vi "F2-alle_sub.vi"(1 "% overtalk D-A":u8, 2 "% overtalk D-T2":u8, 3 "% overtalk D-T1":u8, 4 "binning (s)":refnum<vi>, 5 "Channel Akzeptor":refnum<vi>, 6 "HydraHarp":bool, 7 "Channel Transmitter2":refnum<vi>, 8 "Channel Transmitter1":refnum<vi>, 9 "Channel Donor":refnum<vi>) -> (0 "F2-Values":cluster{dbl, "Value":dbl, dbl[]}[](graph))   [LabVIEW 2009]
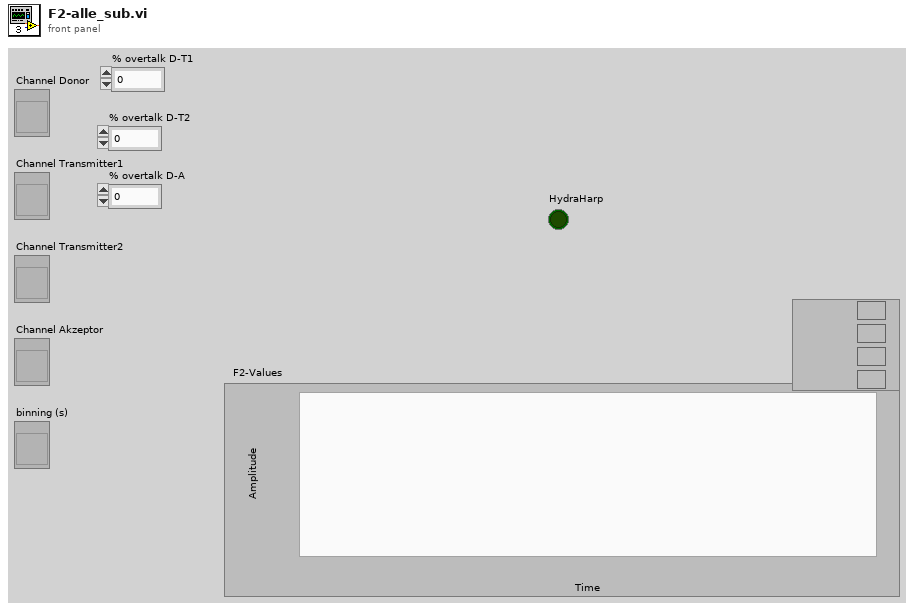
[diagram p1: front panel]
types:
  T1 = cluster{"router channels":u8[], "macro times":dbl[], "micro times":u16[], "invalid times":u32[], "gap times":u32[]}
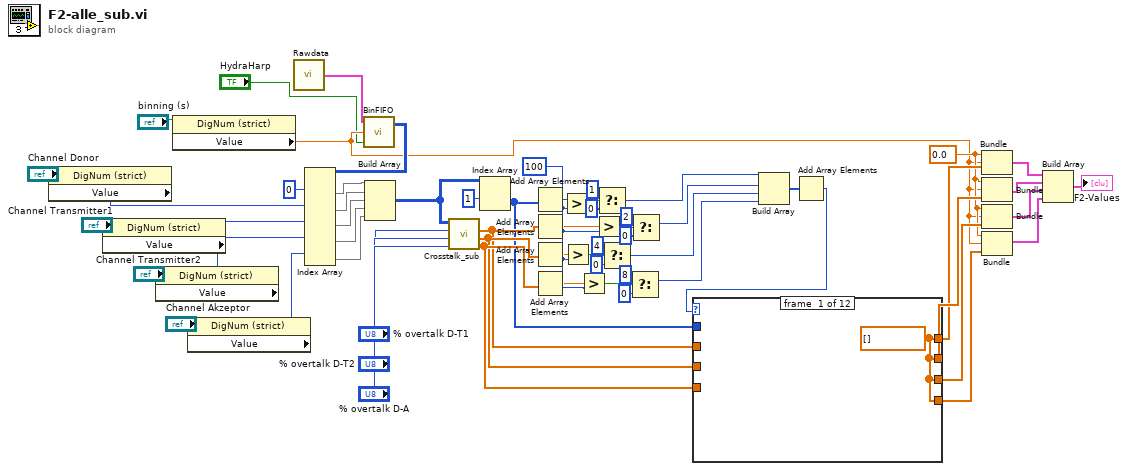
[diagram p0: block diagram]
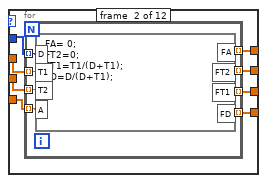
[diagram p2: hidden frame]
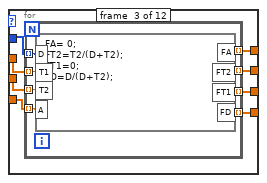
[diagram p3: hidden frame]
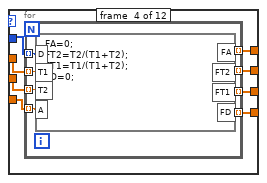
[diagram p4: hidden frame]
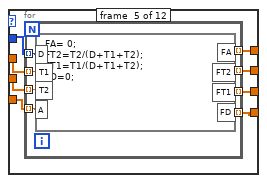
[diagram p5: hidden frame]
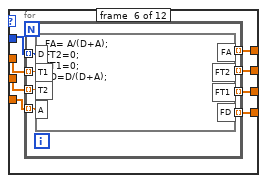
[diagram p6: hidden frame]
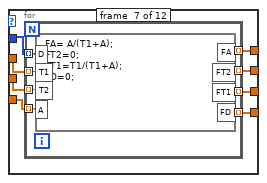
[diagram p7: hidden frame]
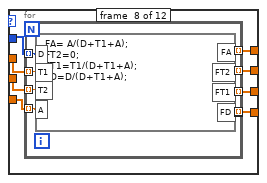
[diagram p8: hidden frame]
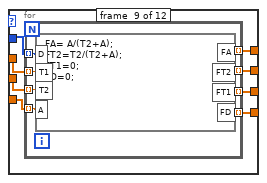
[diagram p9: hidden frame]
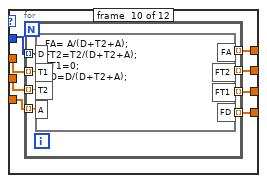
[diagram p10: hidden frame]
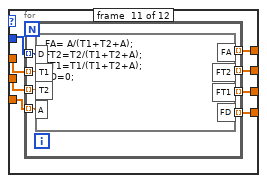
[diagram p11: hidden frame]
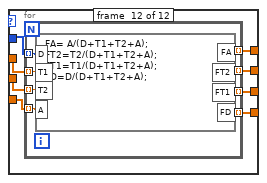
[diagram p12: hidden frame]
diagram:
  w22 = u16 100 ("y")
  w26 = 0.0
  n1 = property on="Property Node" class="DigNum (strict)"(reference="Channel Donor") -> ("Value"=w14:u8)  [unwired: 1 in, 2 out]
  n2 = property on="Property Node" class="DigNum (strict)"(reference="Channel Transmitter1") -> ("Value"=w15:u8)  [unwired: 1 in, 2 out]
  n3 = property on="Property Node" class="DigNum (strict)"(reference="Channel Transmitter2") -> ("Value"=w16:u8)  [unwired: 1 in, 2 out]
  n4 = property on="Property Node" class="DigNum (strict)"(reference="binning (s)") -> ("Value"=w6:dbl)  [unwired: 1 in, 2 out]
  n5 = property on="Property Node" class="DigNum (strict)"(reference="Channel Akzeptor") -> ("Value"=w17:u8)  [unwired: 1 in, 2 out]
  n6 = call "Rawdata.vi"() -> ("output rawdata"=w45:T1)  [unwired: 2 in]
  n7 = call "BinFIFO.vi"("HydraHarp"="HydraHarp", "binning (s)"=w6, "rawdata"=w45) -> ("MCS"=w18:u32[][])  [unwired: 1 out]
  n8 = Index Array(array=w18, index (row) #1=0 ("index (row)"), index (row) #2=w14, index (row) #3=w15, index (row) #4=w16, index (row) #5=w17) -> (element #1=w12:u32[], element #2=w11:u32[], element #3=w10:u32[], element #4=w9:u32[], element #5=w8:u32[])  [unwired: 5 in]
  n9 = Build Array(w12, w11, w10, w9, w8) -> (w7:u32[][])
  n10 = call "Crosstalk_sub.vi"("% overtalk D-T1"="% overtalk D-A", "% overtalk D-T2"="% overtalk D-T2", "% overtalk D-A"="% overtalk D-T1", "MCS_bg_corr"=w7) -> ("Akzeptor"=w5:dbl[], "Transmitter2"=w4:dbl[], "Transmitter1"=w3:dbl[])  [unwired: 1 out]
  n11 = Index Array(array=w7, index (row)=1) -> (element=w2:u32[])  [unwired: 1 in]
  n12 = Add Array Elements(numeric array=w2) -> (sum=w23:u32)
  n13 = Add Array Elements(numeric array=w3) -> (sum=w21:dbl)
  n14 = Add Array Elements(numeric array=w4) -> (sum=w20:dbl)
  n15 = Add Array Elements(numeric array=w5) -> (sum=w19:dbl)
  n16 = Greater?(x=w23, y=w22) -> (0:w44:bool)
  n17 = Greater?(x=w20, y=w22) -> (0:w35:bool)
  n18 = Greater?(x=w19, y=w22) -> (0:w41:bool)
  n19 = Greater?(x=w21, y=w22) -> (0:w38:bool)
  n20 = Select(t=u8 1, s=w44, f=u8 0) -> (s? t:f=w32:u8)
  n21 = Select(t=u8 4, s=w35, f=u8 0) -> (s? t:f=w30:u8)
  n22 = Select(t=u8 8, s=w41, f=u8 0) -> (s? t:f=w29:u8)
  n23 = Select(t=u8 2, s=w38, f=u8 0) -> (s? t:f=w31:u8)
  n24 = Build Array(w32, w31, w30, w29) -> (w28:u8[])
  n25 = Add Array Elements(numeric array=w28) -> (sum=w27:u8)
  n26 = case shown="11" w27 {
    tunnel: w2 -> [_ w70 w86 w102 w118 w134 w150 w166 w182 w198 w214 w230]
    tunnel: w3 -> [_ w69 w85 w101 w117 w133 w149 w165 w181 w197 w213 w229]
    tunnel: w4 -> [_ w68 w84 w100 w116 w132 w148 w164 w180 w196 w212 w228]
    tunnel: w5 -> [_ w67 w83 w99 w115 w131 w147 w163 w179 w195 w211 w227]
    tunnel: [w62 w66 w82 w98 w114 w130 w146 w162 w178 w194 w210 w226] -> w59
    tunnel: [w62 w65 w81 w97 w113 w129 w145 w161 w177 w193 w209 w225] -> w60
    tunnel: [w62 w64 w80 w96 w112 w128 w144 w160 w176 w192 w208 w224] -> w61
    tunnel: [w62 w63 w79 w95 w111 w127 w143 w159 w175 w191 w207 w223] -> w25
    frame #0 {
      w62 = dbl[] []
    }
    frame #1 {
      n27 = for {
        tunnel: w70 -> [w78] mode=indexing
        tunnel: w69 -> [w77] mode=indexing
        tunnel: w68 -> [w76] mode=indexing
        tunnel: w67 -> [w75] mode=indexing
        tunnel: [w74] -> w66 mode=indexing
        tunnel: [w73] -> w65 mode=indexing
        tunnel: [w72] -> w64 mode=indexing
        tunnel: [w71] -> w63 mode=indexing
        n28 = formula code="FA= 0;\nFT2=0;\nFT1=T1/(D+T1);\nFD=D/(D+T1);"("D"=w78, "T1"=w77, "T2"=w76, "A"=w75) -> ("FA"=w74:dbl, "FT2"=w73:dbl, "FT1"=w72:dbl, "FD"=w71:dbl)
      }
    }
    frame #2 {
      n29 = for {
        tunnel: w86 -> [w94] mode=indexing
        tunnel: w85 -> [w93] mode=indexing
        tunnel: w84 -> [w92] mode=indexing
        tunnel: w83 -> [w91] mode=indexing
        tunnel: [w90] -> w82 mode=indexing
        tunnel: [w89] -> w81 mode=indexing
        tunnel: [w88] -> w80 mode=indexing
        tunnel: [w87] -> w79 mode=indexing
        n30 = formula code="FA= 0;\nFT2=T2/(D+T2);\nFT1=0;\nFD=D/(D+T2);"("D"=w94, "T1"=w93, "T2"=w92, "A"=w91) -> ("FA"=w90:dbl, "FT2"=w89:dbl, "FT1"=w88:dbl, "FD"=w87:dbl)
      }
    }
    frame #3 {
      n31 = for {
        tunnel: w102 -> [w110] mode=indexing
        tunnel: w101 -> [w109] mode=indexing
        tunnel: w100 -> [w108] mode=indexing
        tunnel: w99 -> [w107] mode=indexing
        tunnel: [w106] -> w98 mode=indexing
        tunnel: [w105] -> w97 mode=indexing
        tunnel: [w104] -> w96 mode=indexing
        tunnel: [w103] -> w95 mode=indexing
        n32 = formula code="FA=0;\nFT2=T2/(T1+T2);\nFT1=T1/(T1+T2);\nFD=0;"("D"=w110, "T1"=w109, "T2"=w108, "A"=w107) -> ("FA"=w106:dbl, "FT2"=w105:dbl, "FT1"=w104:dbl, "FD"=w103:dbl)
      }
    }
    frame #4 {
      n33 = for {
        tunnel: w118 -> [w126] mode=indexing
        tunnel: w117 -> [w125] mode=indexing
        tunnel: w116 -> [w124] mode=indexing
        tunnel: w115 -> [w123] mode=indexing
        tunnel: [w122] -> w114 mode=indexing
        tunnel: [w121] -> w113 mode=indexing
        tunnel: [w120] -> w112 mode=indexing
        tunnel: [w119] -> w111 mode=indexing
        n34 = formula code="FA= 0;\nFT2=T2/(D+T1+T2);\nFT1=T1/(D+T1+T2);\nFD=0;"("D"=w126, "T1"=w125, "T2"=w124, "A"=w123) -> ("FA"=w122:dbl, "FT2"=w121:dbl, "FT1"=w120:dbl, "FD"=w119:dbl)
      }
    }
    frame #5 {
      n35 = for {
        tunnel: w134 -> [w142] mode=indexing
        tunnel: w133 -> [w141] mode=indexing
        tunnel: w132 -> [w140] mode=indexing
        tunnel: w131 -> [w139] mode=indexing
        tunnel: [w138] -> w130 mode=indexing
        tunnel: [w137] -> w129 mode=indexing
        tunnel: [w136] -> w128 mode=indexing
        tunnel: [w135] -> w127 mode=indexing
        n36 = formula code="FA= A/(D+A);\nFT2=0;\nFT1=0;\nFD=D/(D+A);"("D"=w142, "T1"=w141, "T2"=w140, "A"=w139) -> ("FA"=w138:dbl, "FT2"=w137:dbl, "FT1"=w136:dbl, "FD"=w135:dbl)
      }
    }
    frame #6 {
      n37 = for {
        tunnel: w150 -> [w158] mode=indexing
        tunnel: w149 -> [w157] mode=indexing
        tunnel: w148 -> [w156] mode=indexing
        tunnel: w147 -> [w155] mode=indexing
        tunnel: [w154] -> w146 mode=indexing
        tunnel: [w153] -> w145 mode=indexing
        tunnel: [w152] -> w144 mode=indexing
        tunnel: [w151] -> w143 mode=indexing
        n38 = formula code="FA= A/(T1+A);\nFT2=0;\nFT1=T1/(T1+A);\nFD=0;"("D"=w158, "T1"=w157, "T2"=w156, "A"=w155) -> ("FA"=w154:dbl, "FT2"=w153:dbl, "FT1"=w152:dbl, "FD"=w151:dbl)
      }
    }
    frame #7 {
      n39 = for {
        tunnel: w166 -> [w174] mode=indexing
        tunnel: w165 -> [w173] mode=indexing
        tunnel: w164 -> [w172] mode=indexing
        tunnel: w163 -> [w171] mode=indexing
        tunnel: [w170] -> w162 mode=indexing
        tunnel: [w169] -> w161 mode=indexing
        tunnel: [w168] -> w160 mode=indexing
        tunnel: [w167] -> _ mode=indexing
        tunnel: [w167] -> w159 mode=indexing
        n40 = formula code="FA= A/(D+T1+A);\nFT2=0;\nFT1=T1/(D+T1+A);\nFD=D/(D+T1+A);"("D"=w174, "T1"=w173, "T2"=w172, "A"=w171) -> ("FA"=w170:dbl, "FT2"=w169:dbl, "FT1"=w168:dbl, "FD"=w167:dbl)
      }
    }
    frame #8 {
      n41 = for {
        tunnel: w182 -> [w190] mode=indexing
        tunnel: w181 -> [w189] mode=indexing
        tunnel: w180 -> [w188] mode=indexing
        tunnel: w179 -> [w187] mode=indexing
        tunnel: [w186] -> w178 mode=indexing
        tunnel: [w185] -> w177 mode=indexing
        tunnel: [w184] -> w176 mode=indexing
        tunnel: [w183] -> w175 mode=indexing
        n42 = formula code="FA= A/(T2+A);\nFT2=T2/(T2+A);\nFT1=0;\nFD=0;"("D"=w190, "T1"=w189, "T2"=w188, "A"=w187) -> ("FA"=w186:dbl, "FT2"=w185:dbl, "FT1"=w184:dbl, "FD"=w183:dbl)
      }
    }
    frame #9 {
      n43 = for {
        tunnel: w198 -> [w206] mode=indexing
        tunnel: w197 -> [w205] mode=indexing
        tunnel: w196 -> [w204] mode=indexing
        tunnel: w195 -> [w203] mode=indexing
        tunnel: [w202] -> w194 mode=indexing
        tunnel: [w201] -> w193 mode=indexing
        tunnel: [w200] -> w192 mode=indexing
        tunnel: [w199] -> w191 mode=indexing
        n44 = formula code="FA= A/(D+T2+A);\nFT2=T2/(D+T2+A);\nFT1=0;\nFD=D/(D+T2+A);"("D"=w206, "T1"=w205, "T2"=w204, "A"=w203) -> ("FA"=w202:dbl, "FT2"=w201:dbl, "FT1"=w200:dbl, "FD"=w199:dbl)
      }
    }
    frame #10 {
      n45 = for {
        tunnel: w214 -> [w222] mode=indexing
        tunnel: w213 -> [w221] mode=indexing
        tunnel: w212 -> [w220] mode=indexing
        tunnel: w211 -> [w219] mode=indexing
        tunnel: [w218] -> w210 mode=indexing
        tunnel: [w217] -> w209 mode=indexing
        tunnel: [w216] -> w208 mode=indexing
        tunnel: [w215] -> w207 mode=indexing
        n46 = formula code="FA= A/(T1+T2+A);\nFT2=T2/(T1+T2+A);\nFT1=T1/(T1+T2+A);\nFD=0;"("D"=w222, "T1"=w221, "T2"=w220, "A"=w219) -> ("FA"=w218:dbl, "FT2"=w217:dbl, "FT1"=w216:dbl, "FD"=w215:dbl)
      }
    }
    frame #11 {
      n47 = for {
        tunnel: w230 -> [w238] mode=indexing
        tunnel: w229 -> [w237] mode=indexing
        tunnel: w228 -> [w236] mode=indexing
        tunnel: w227 -> [w235] mode=indexing
        tunnel: [w234] -> w226 mode=indexing
        tunnel: [w233] -> w225 mode=indexing
        tunnel: [w232] -> w224 mode=indexing
        tunnel: [w231] -> w223 mode=indexing
        n48 = formula code="FA= A/(D+T1+T2+A);\nFT2=T2/(D+T1+T2+A);\nFT1=T1/(D+T1+T2+A);\nFD=D/(D+T1+T2+A);"("D"=w238, "T1"=w237, "T2"=w236, "A"=w235) -> ("FA"=w234:dbl, "FT2"=w233:dbl, "FT1"=w232:dbl, "FD"=w231:dbl)
      }
    }
  }
  n49 = Bundle(w26, "Value"=w6, w59) -> (w49:cluster{dbl, "Value":dbl, dbl[]})  [unwired: 1 in]
  n50 = Bundle(w26, "Value"=w6, w60) -> (w48:cluster{dbl, "Value":dbl, dbl[]})  [unwired: 1 in]
  n51 = Bundle(w26, "Value"=w6, w61) -> (w47:cluster{dbl, "Value":dbl, dbl[]})  [unwired: 1 in]
  n52 = Bundle(w26, "Value"=w6, w25) -> (w24:cluster{dbl, "Value":dbl, dbl[]})  [unwired: 1 in]
  n53 = Build Array(w49, w48, w47, w24) -> (→"F2-Values":cluster{dbl, "Value":dbl, dbl[]}[])
